vi "integer7_overlayDraw.vi"() -> ()   [LabVIEW 2018]
uses:
  <vilib>/userdefined/High Color/IMAQdx.ctl
  <vilib>/vision/driver/NI_Vision_Acquisition_Software.lvlib
panel:
  out "Image":T1(plugin-control)
  in  "停止":bool
  out "error out":errorcluster
  out "大小":i32
  in  "距离阈值":dbl=1000.0 format="%#_13g"
  in  "角度阈值":dbl=30.0 format="%#_13g"
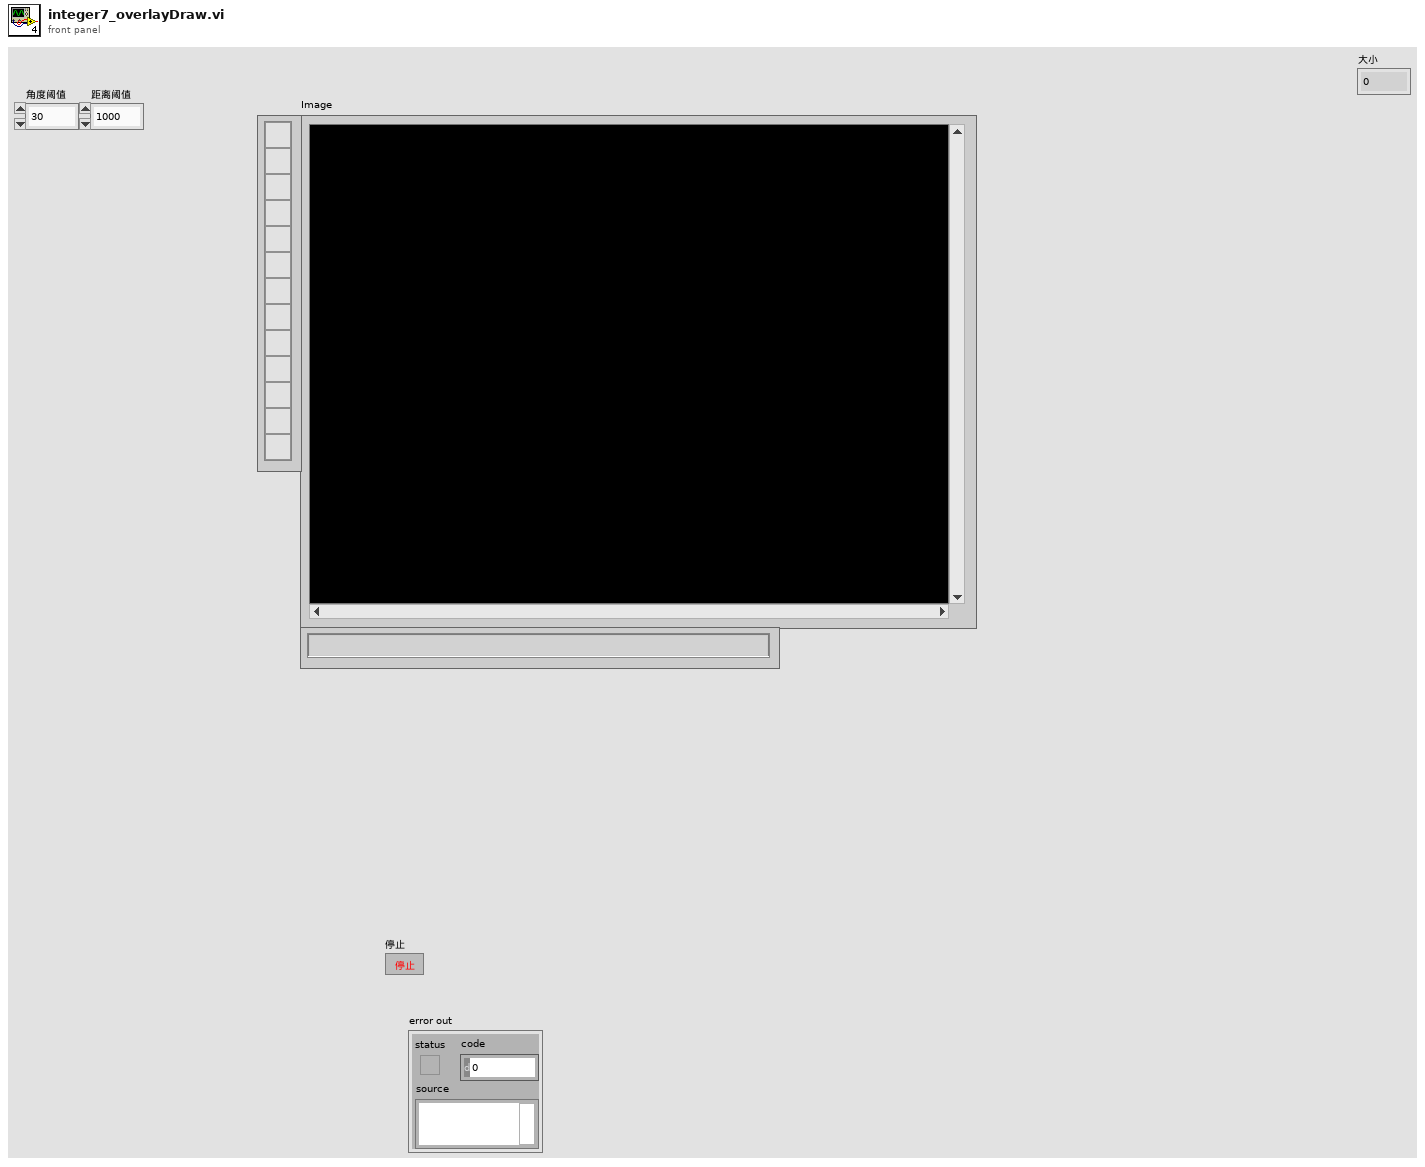
[diagram p1: front panel]
types:
  T1 = typedef "IMAQ Image.ctl" = refnum<image>
  T2 = typedef "IMAQdx.ctl" = refnum<k21>
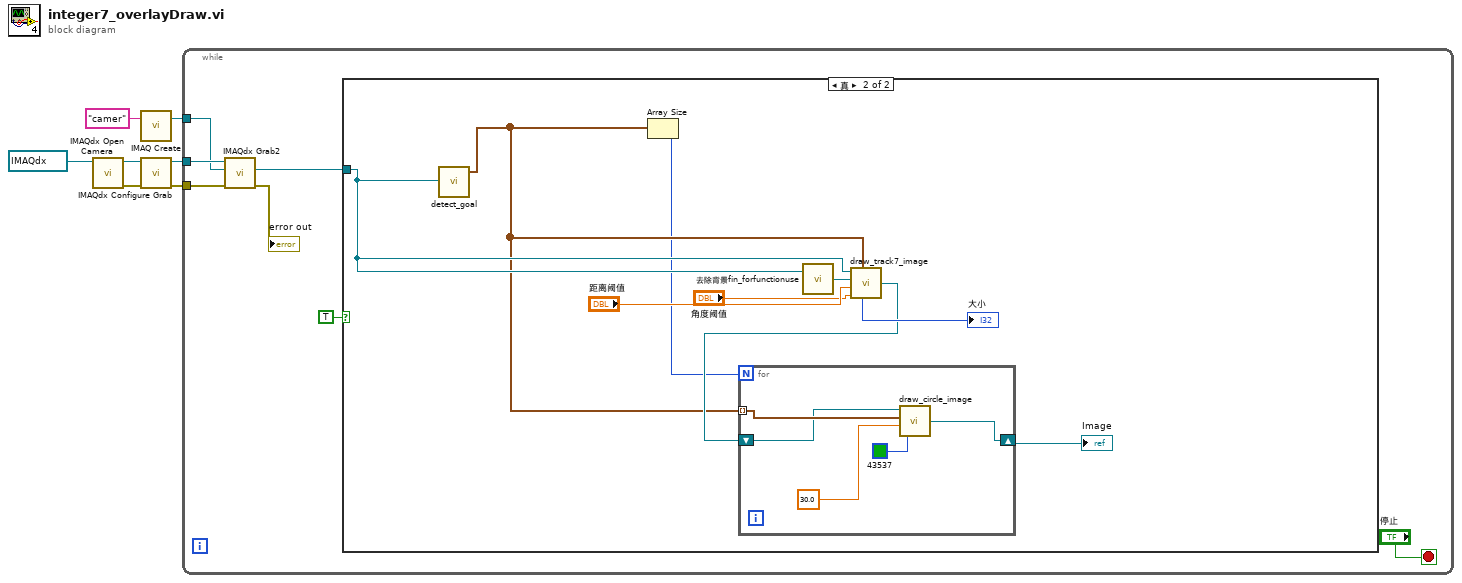
[diagram p0: block diagram]
diagram:
  n1 = call <vilib>:"IMAQdx Open Camera.vi"("Session In"=T2 "cam2") -> ("error out"=w6:errorcluster, "Session Out"=w7:T2)  [unwired: 9 in]
  n2 = call "IMAQ Create"("Image Name"="camer") -> ("New Image"=w4:T1)  [unwired: 4 in, 1 out]
  n3 = call <vilib>:"IMAQdx Configure Grab.vi"("error in"=w6, "Session In"=w7) -> ("error out"=w1:errorcluster, "Session Out"=w5:T2)  [unwired: 8 in]
  n4 = while {
    tunnel: w5 -> [w14]
    tunnel: w4 -> [w13]
    tunnel: w1 -> [w11]
    stop <- "停止" stop-if-true
    n5 = call <vilib>:"IMAQdx Grab2.vi"("error in"=w11, "Image In"=w13, "Session In"=w14) -> ("error out"=→"error out":errorcluster, "Image Out"=w9:T1)  [unwired: 5 in, 2 out]
    n6 = case shown="真" TRUE {
      tunnel: w9 -> [_ w18]
      frame False {
      }
      frame True {
        n7 = call "detect_goal.vi"("Image Out"=w18) -> ("goal_pos"=w17:cluster{"ave x":dbl, "ave y":dbl}[])  [unwired: 2 out]
        n8 = Array Size(array=w17) -> (size(s)=w15:i32)
        n9 = call "去除背景fin_forfunctionuse.vi"("Image Src"=w18) -> ("Image Out"=w19:T1)  [unwired: 1 in]
        n10 = call "draw_track7_image.vi"("GOALpos"=w17, "角度阈值"="角度阈值", "距离阈值"="距离阈值", "bin_billard"=w19, "color_billard"=w18) -> ("color_billard 2"=w22:T1, "大小"=→"大小":i32)
        n11 = for {
          N: w15 -> [_]
          tunnel: w17 -> [w27] mode=indexing
          shift-right: [w24] -> w16
          shift-left: w22 -> [w25]
          n12 = call "draw_circle_image.vi"("Color"=u32 43537 ("color(black)"), "radius"=30.0, "Position"=w27, "Image"=w25) -> ("Image Out"=w24:T1)
        }
        "Image" <- w16
      }
    }
  }
